vi "accuracy.vi"(1 "Y_actual":dbl[][](array[numeric]), 2 "Y_predicted":dbl[][](array[numeric])) -> (0 "Accuracy":dbl)   [LabVIEW 2020]
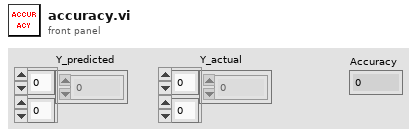
[diagram p1: front panel]
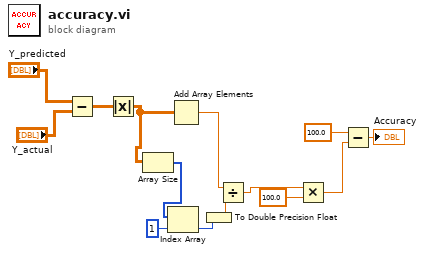
[diagram p0: block diagram]
diagram:
  n1 = Subtract(x="Y_predicted", y="Y_actual") -> (x-y=w14:dbl[][])
  n2 = Absolute Value(x=w14) -> (abs(x)=w13:dbl[][])
  n3 = Array Size(array=w13) -> (size(s)=w12:i32[])
  n4 = Index Array(array=w12, index=1) -> (element=w10:i32)
  n5 = Add Array Elements(numeric array=w13) -> (sum=w1:dbl)
  n6 = To Double Precision Float(number=w10) -> (double precision float=w9:dbl)
  n7 = Divide(x=w1, y=w9) -> (x/y=w8:dbl)
  n8 = Multiply(x=w8, y=100.0) -> (x*y=w6:dbl)
  n9 = Subtract(x=100.0, y=w6) -> (x-y=→"Accuracy":dbl)
